vi "image2variant.vi"(10 "image_1d":sgl[](array[numeric]), 11 "Data":T1 {"slice orientation" items=["transverse unflipped", "coronal unflipped", "sagittal unflipped", "transverse flipped", "coronal flipped", "sagittal flipped"]}) -> (2 "variant":variant)   [LabVIEW 2014]
uses:
  control/head_data.ctl
  image2data_2d.vi
  image2data_3d.vi
  image2data_4d.vi
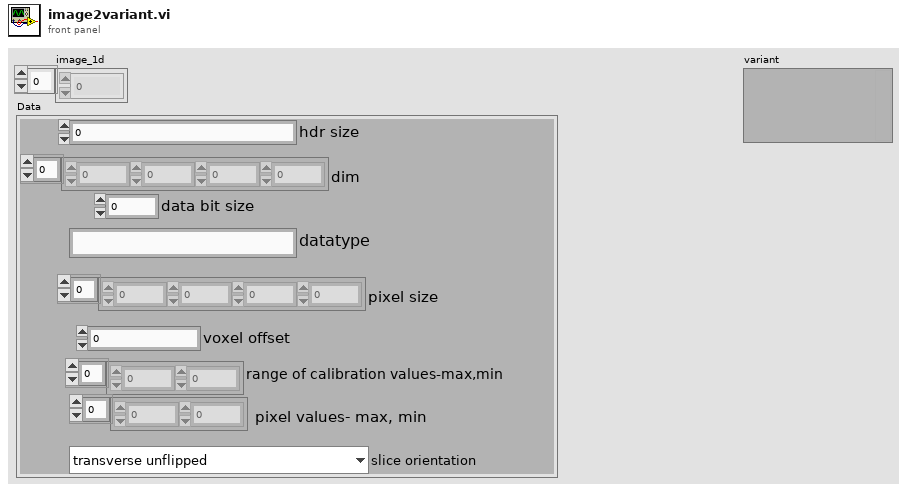
[diagram p1: front panel]
types:
  T1 = typedef "head_data.ctl" = cluster{"hdr size":i32, "dim":i32[], "data bit size":i32, "datatype":string, "pixel size ":sgl[], "voxel offset":sgl, "range of calibration values-max,min":sgl[], " pixel values- max, min":sgl[], "slice orientation":u16}
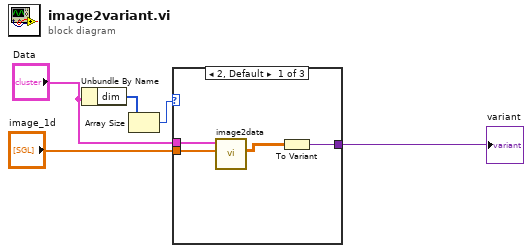
[diagram p0: block diagram]
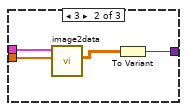
[diagram p2: hidden frame]
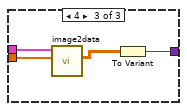
[diagram p3: hidden frame]
diagram:
  n1 = Unbundle By Name("Data") -> ("dim"=w3:i32[])
  n2 = Array Size(array=w3) -> (size(s)=w2:i32)
  n3 = case shown="2, Default" w2 {
    tunnel: "image_1d" -> [w9 w13 w17]
    tunnel: "Data" -> [w8 w12 w16]
    tunnel: [w6 w10 w14] -> w1
    frame 2, Default {
      n4 = call-poly "image2data.vi"("image_1d"=w9, "Data"=w8) -> ("imag2_2d"=w7:sgl[][])  [unwired: 8 in, 1 out]
      n5 = To Variant(anything=w7) -> (Variant=w6:variant)
    }
    frame 3 {
      n6 = call-poly "image2data.vi"("image_1d"=w13, "Data"=w12) -> ("imag3_3d"=w11:sgl[][][])  [unwired: 8 in, 1 out]
      n7 = To Variant(anything=w11) -> (Variant=w10:variant)
    }
    frame 4 {
      n8 = call-poly "image2data.vi"("image_1d"=w17, "Data"=w16) -> ("image_4d"=w15:sgl[][][][])  [unwired: 8 in, 1 out]
      n9 = To Variant(anything=w15) -> (Variant=w14:variant)
    }
  }
  "variant" <- w1
